vi "Eat Whitespace.vi"(8 "Error In":errorcluster, 11 "Parser In":refnum<class "Parser.lvclass">) -> (0 "Error Out":errorcluster, 3 "Parser Out":refnum<class "Parser.lvclass">)   [LabVIEW 2017, in "Mustache.lvlib" / "Parser.lvclass"]
uses:
  Parser.lvclass
  Parser.lvclass/Parser.ctl
  <vilib>/Utility/error.llb/whitespace.ctl
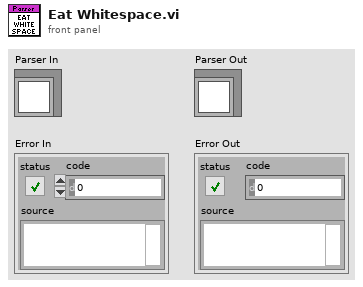
[diagram p1: front panel]
types:
  T1 = typedef "Mustache.lvlib/Parser.lvclass/Token Class.ctl" = enum16{"Normal", "Stand Alone", "Whitespace"}
  T2 = typedef "Mustache.lvlib/Parser.lvclass/Token.ctl" = cluster{"Type":T3, "Data":variant}
  T3 = typedef "Mustache.lvlib/Parser.lvclass/Token Types.ctl" = enum16{"Text", "Escaped Tag", "Unescaped Tag", "Section", "Incomplete Section", "Partial"}
  T4 = typedef "whitespace.ctl" = u16
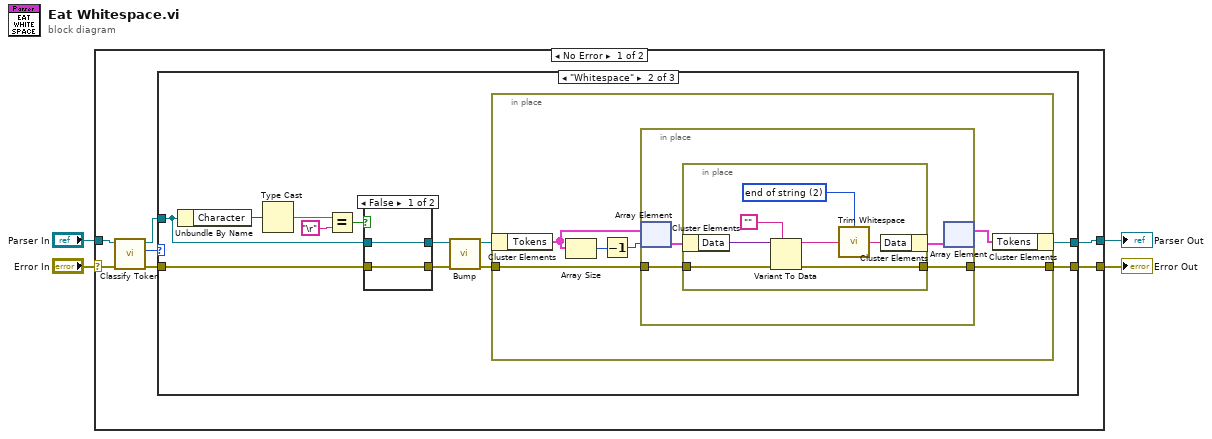
[diagram p0: block diagram]
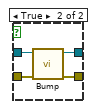
[diagram p3: hidden frame]
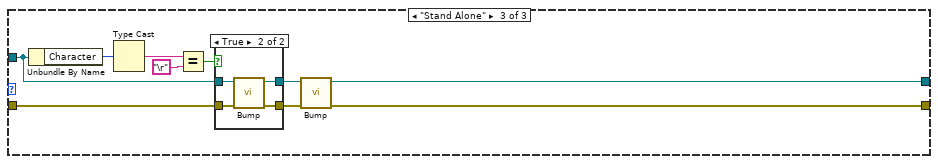
[diagram p4: hidden frame]
diagram:
  n1 = case shown="No Error" "Error In" {
    selector: "Error In" -> [w10 w65]
    tunnel: "Parser In" -> [w11 w66]
    tunnel: [w5 w66] -> w2
    tunnel: [w6 w65] -> w1
    frame No Error {
      n2 = call "Classify Token.vi"("Error In"=w10, "Parser In"=w11) -> ("Error Out"=w7:errorcluster, "Class"=w9:T1, "Parser Out"=w8:refnum<class "Parser.lvclass">)  [unwired: 7 in]
      n3 = case shown="\"Whitespace\"" w9 {
        tunnel: w8 -> [w13 w21 w54]
        tunnel: w7 -> [w12 w20 w55]
        tunnel: [w12 w14 w50] -> w6
        tunnel: [w13 w16 w49] -> w5
        frame "Normal", Default {
        }
        frame "Whitespace" {
          n4 = Unbundle By Name(w21) -> ("Character"=w25:u8)
          n5 = Type Cast(x=w25) -> (*(type *) &x=w24:string)  [unwired: 1 in]
          n6 = Equal?(x=w24, y="\r") -> (x = y?=w22:bool)
          n7 = case shown="False" w22 {
            tunnel: w21 -> [w44 w48]
            tunnel: [w44 w47] -> w19
            tunnel: w20 -> [w43 w46]
            tunnel: [w43 w45] -> w18
            frame False {
            }
            frame True {
              n8 = call "Bump.vi"("Error In"=w46, "Parser In"=w48) -> ("Error Out"=w45:errorcluster, "Parser Out"=w47:refnum<class "Parser.lvclass">)  [unwired: 8 in]
            }
          }
          n9 = call "Bump.vi"("Error In"=w18, "Parser In"=w19) -> ("Error Out"=w15:errorcluster, "Parser Out"=w17:refnum<class "Parser.lvclass">)  [unwired: 8 in]
          n10 = in-place {
            in-place-border: w15 -> [w27]
            in-place-border: [w26] -> w14
            n11 = in-place-cluster #1(w17) -> ("Tokens"=w30:T2[])
            n12 = Array Size(array=w30) -> (size(s)=w29:i32)
            n13 = Decrement(x=w29) -> (x-1=w28:i32)
            n14 = in-place {
              in-place-border: w27 -> [w33]
              in-place-border: [w32] -> w26
              n15 = in-place-array #2(w30, w28) -> (w35:T2)
              n16 = in-place {
                in-place-border: w33 -> [w41]
                in-place-border: [w40] -> w32
                w38 = T4 2 items=["both", "start of string", "end of string"] ("location (both)")
                n17 = in-place-cluster #3(w35) -> ("Data"=w42:variant)
                n18 = Variant To Data(error in=w41, type="", Variant=w42) -> (data=w37:string, error out=w40:errorcluster)
                n19 = call <vilib>:"Trim Whitespace.vi"("string"=w37, "location (both)"=w38) -> ("trimmed string"=w36:string)
                n20 = in-place-cluster #3("Data"=w36) -> (w34:T2)
              }
              n21 = in-place-array #2(w34) -> (w31:T2[])  [unwired: 1 out]
            }
            n22 = in-place-cluster #1("Tokens"=w31) -> (w16:refnum<class "Parser.lvclass">)
          }
        }
        frame "Stand Alone" {
          n23 = Unbundle By Name(w54) -> ("Character"=w58:u8)
          n24 = Type Cast(x=w58) -> (*(type *) &x=w57:string)  [unwired: 1 in]
          n25 = Equal?(x=w57, y="\r") -> (x = y?=w53:bool)
          n26 = case shown="True" w53 {
            tunnel: w55 -> [w59 w64]
            tunnel: w54 -> [w60 w63]
            tunnel: [w60 w62] -> w52
            tunnel: [w59 w61] -> w51
            frame False {
            }
            frame True {
              n27 = call "Bump.vi"("Error In"=w64, "Parser In"=w63) -> ("Error Out"=w61:errorcluster, "Parser Out"=w62:refnum<class "Parser.lvclass">)  [unwired: 8 in]
            }
          }
          n28 = call "Bump.vi"("Error In"=w51, "Parser In"=w52) -> ("Error Out"=w50:errorcluster, "Parser Out"=w49:refnum<class "Parser.lvclass">)  [unwired: 8 in]
        }
      }
    }
    frame Error {
    }
  }
  "Parser Out" <- w2
  "Error Out" <- w1
